vi "Next Step.vi"(8 "error in (no error)":errorcluster, 11 "Double Scanner in":refnum<class "Double Scanner.lvclass">) -> (0 "error out":errorcluster, 1 "Current Step":u32, 2 "Current Position":dbl, 3 "Double Scanner out":refnum<class "Double Scanner.lvclass">)   [LabVIEW 2017, in "Double Scanner.lvclass"]
doc: "(Dynamic) Move to the next preconfigured step of this Scanner, and return the current position (actual, not intended) of this Scanner. Increment the step counter by one."
uses:
  Double Scanner.lvclass
  Double Scanner.lvclass/Double Scanner.ctl
  Scanner/Scanner.lvclass
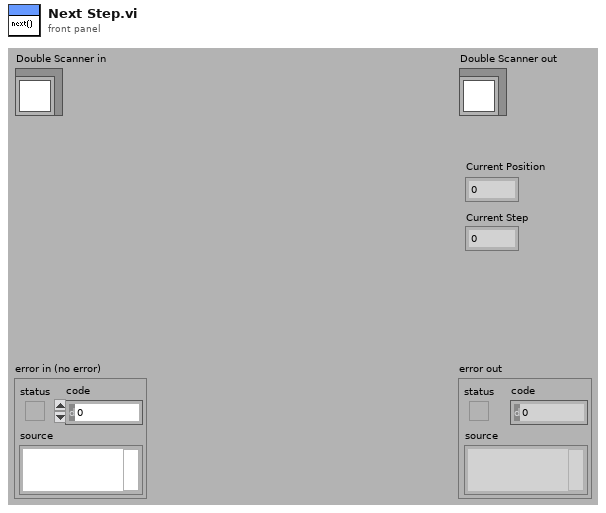
[diagram p1: front panel]
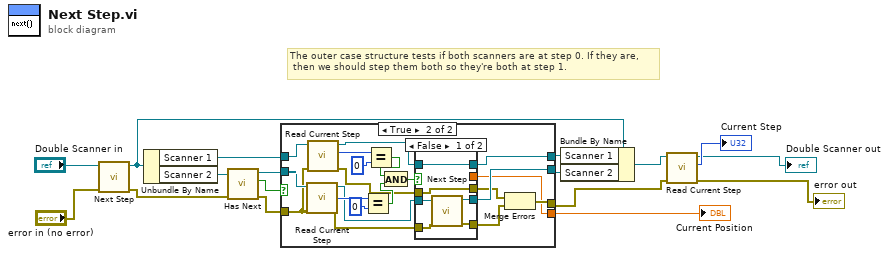
[diagram p0: block diagram]
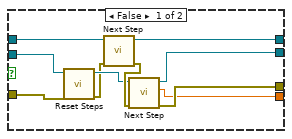
[diagram p2: hidden frame]
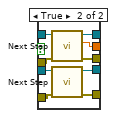
[diagram p3: hidden frame]
diagram:
  # "The outer case structure tests if both scanners are at step 0. If they are,\n then we should step them both so they're both at step 1."
  n1 = call-parent "Next Step.vi"("error in (no error)"="error in (no error)", "Scanner in"="Double Scanner in") -> ("error out"=w12:errorcluster, "Scanner out"=w9:refnum<class "Double Scanner.lvclass">)  [unwired: 8 out]
  n2 = Unbundle By Name(w9) -> ("Scanner 1"=w14:refnum<class "Scanner.lvclass">, "Scanner 2"=w17:refnum<class "Scanner.lvclass">)
  n3 = call-dynamic "Has Next.vi"("error in (no error)"=w12, "Scanner.lvclass in"=w17) -> ("error out"=w13:errorcluster, "Again?"=w16:bool, "Scanner.lvclass out"=w15:refnum<class "Scanner.lvclass">)  [unwired: 7 in]
  n4 = case shown="True" w16 {
    tunnel: w15 -> [w18 w46]
    tunnel: w13 -> [w20 w45]
    tunnel: [w23 w29] -> w3
    tunnel: [w24 w33] -> w7
    tunnel: w14 -> [w27 w47]
    tunnel: [w26 w32] -> w8
    tunnel: [w22 w28] -> w1
    frame False {
      n5 = call-dynamic "Reset Steps.vi"("error in (no error)"=w20, "Scanner in"=w18) -> ("error out"=w19:errorcluster, "Scanner out"=w21:refnum<class "Scanner.lvclass">)  [unwired: 8 in]
      n6 = call-dynamic "Next Step.vi"("error in (no error)"=w19, "Scanner in"=w27) -> ("error out"=w25:errorcluster, "Scanner out"=w26:refnum<class "Scanner.lvclass">)  [unwired: 6 in, 2 out]
      n7 = call-dynamic "Next Step.vi"("error in (no error)"=w25, "Scanner in"=w21) -> ("error out"=w23:errorcluster, "Current Position"=w22:dbl, "Scanner out"=w24:refnum<class "Scanner.lvclass">)  [unwired: 6 in, 1 out]
    }
    frame True {
      n8 = call-dynamic "Read Current Step.vi"("error in (no error)"=w45, "Scanner.lvclass in"=w46) -> ("error out"=w35:errorcluster, "Current Step"=w42:u32, "Scanner.lvclass out"=w36:refnum<class "Scanner.lvclass">)  [unwired: 5 in, 2 out]
      n9 = call-dynamic "Read Current Step.vi"("error in (no error)"=w45, "Scanner.lvclass in"=w47) -> ("error out"=w34:errorcluster, "Current Step"=w44:u32, "Scanner.lvclass out"=w37:refnum<class "Scanner.lvclass">)  [unwired: 5 in, 2 out]
      n10 = Equal?(x=w42, y=u32 0) -> (x = y?=w39:bool)
      n11 = Equal?(x=w44, y=u32 0) -> (x = y?=w40:bool)
      n12 = And(x=w40, y=w39) -> (x .and. y?=w38:bool)
      n13 = case shown="False" w38 {
        tunnel: w37 -> [w52 w62]
        tunnel: w36 -> [w53 w61]
        tunnel: w35 -> [w49 w60]
        tunnel: w34 -> [w48 w59]
        tunnel: [w51 w57] -> w33
        tunnel: [w52 w58] -> w32
        tunnel: [w48 w56] -> w31
        tunnel: [w50 w55] -> w30
        tunnel: [_ w54] -> w28
        frame False {
          n14 = call-dynamic "Next Step.vi"("error in (no error)"=w49, "Scanner in"=w53) -> ("error out"=w50:errorcluster, "Scanner out"=w51:refnum<class "Scanner.lvclass">)  [unwired: 6 in, 2 out]
        }
        frame True {
          n15 = call-dynamic "Next Step.vi"("error in (no error)"=w59, "Scanner in"=w62) -> ("error out"=w56:errorcluster, "Current Position"=w54:dbl, "Scanner out"=w58:refnum<class "Scanner.lvclass">)  [unwired: 6 in, 1 out]
          n16 = call-dynamic "Next Step.vi"("error in (no error)"=w60, "Scanner in"=w61) -> ("error out"=w55:errorcluster, "Scanner out"=w57:refnum<class "Scanner.lvclass">)  [unwired: 6 in, 2 out]
        }
      }
      n17 = Merge Errors(w31, w30) -> (w29:errorcluster)
    }
  }
  "Current Position" <- w1
  n18 = Bundle By Name(cluster=w9, "Scanner 1"=w8, "Scanner 2"=w7) -> (w6:refnum<class "Double Scanner.lvclass">)
  n19 = call-dynamic "Read Current Step.vi"("error in (no error)"=w3, "Double Scanner in"=w6) -> ("error out"=→"error out":errorcluster, "Current step"=→"Current Step":u32, "Double Scanner out"=→"Double Scanner out":refnum<class "Double Scanner.lvclass">)  [unwired: 5 in, 2 out]
